vi "Rod Control.vi"(6 "Time (s)":dbl, 9 "Rod Height (cm) in":dbl, 10 "Shim Out":bool, 11 "Shim In":bool) -> (2 "Change in Reactivity":dbl, 3 "Rod Height (cm) out":dbl)   [LabVIEW 2019]
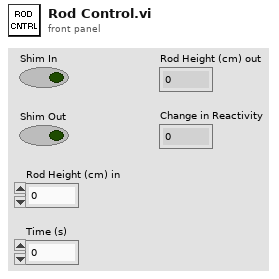
[diagram p1: front panel]
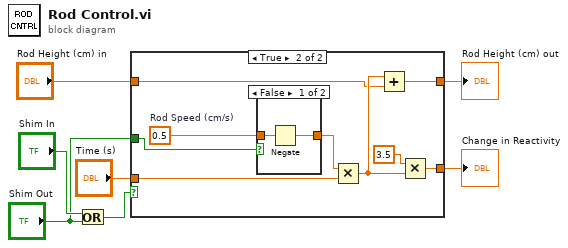
[diagram p0: block diagram]
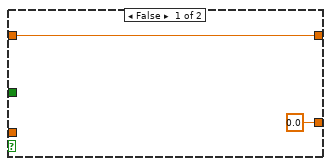
[diagram p2: hidden frame]
diagram:
  n1 = Or(x="Shim In", y="Shim Out") -> (x .or. y?=w4:bool)
  n2 = case shown="True" w4 {
    tunnel: [0.0 w13] -> w5
    tunnel: "Time (s)" -> [_ w17]
    tunnel: "Shim Out" -> [_ w16]
    tunnel: "Rod Height (cm) in" -> [w8 w11]
    tunnel: [w8 w10] -> w7
    frame False {
    }
    frame True {
      w18 = 0.5  # Rod Speed (cm/s)
      n3 = case shown="False" w16 {
        tunnel: w18 -> [w20 w21]
        tunnel: [w19 w21] -> w14
        frame False {
          n4 = Negate(x=w20) -> (-x=w19:dbl)
        }
        frame True {
        }
      }
      n5 = Multiply(x=w14, y=w17) -> (x*y=w12:dbl)
      n6 = Add(x=w12, y=w11) -> (x+y=w10:dbl)
      n7 = Multiply(x=3.5, y=w12) -> (x*y=w13:dbl)
    }
  }
  "Rod Height (cm) out" <- w7
  "Change in Reactivity" <- w5
